vi "Generator.GetEvents.vi"(8 "error in (no error)":errorcluster, 11 "Generator in":refnum<class "Generator.lvclass">) -> (0 "error out":errorcluster, 3 "Generator":cluster{"Public Events":T1, "Public Events":T2})   [LabVIEW 2019, in "Generator.lvclass"]
uses:
  Generator.lvclass
  <vilib>/JKI/JKI SMO/SMO/SMO.lvclass
  Typedefs/PublicEvents--Generator.getGeneratorWaveforms.ctl
  Typedefs/PublicEvents--Cluster.ctl
  <vilib>/JKI/JKI SMO/SMO/Typedefs/Reserve State--Enum.ctl
  <vilib>/JKI/JKI SMO/SMO/Typedefs/SMOState --Enum.ctl
  <vilib>/JKI/JKI SMO/SMO/Typedefs/Public Events.ctl
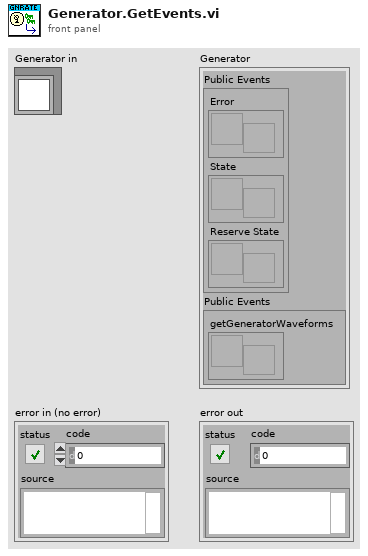
[diagram p1: front panel]
types:
  T1 = typedef "SMO.lvclass/Public Events.ctl" = cluster{"Error":refnum<user-event>, "State":refnum<user-event>, "Reserve State":refnum<user-event>}
  T2 = typedef "Generator.lvclass/PublicEvents--Cluster.ctl" = cluster{"getGeneratorWaveforms":refnum<user-event>}
  T3 = cluster{"Public Events":T1, "Generator.Public Events":T2}
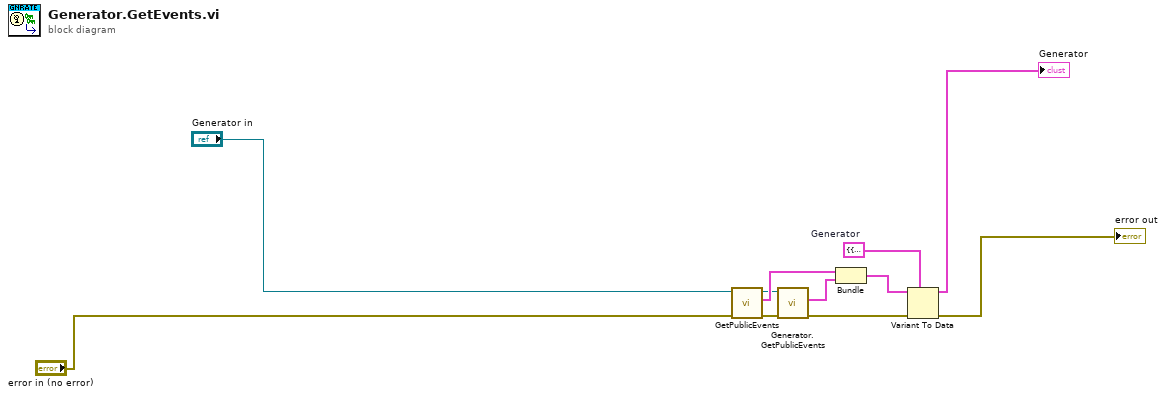
[diagram p0: block diagram]
diagram:
  w8 = cluster{"Public Events":T1, "Public Events":T2} {"Public Events"={"Error"=refnum, "State"=refnum, "Reserve State"=refnum}, "Public Events"={"getGeneratorWaveforms"=refnum}}  # Generator
  n1 = call <vilib>:"GetPublicEvents.vi"("error in (no error)"="error in (no error)", "SMO"="Generator in") -> ("error out"=w4:errorcluster, "Public Events"=w3:T1, "SMO out"=w1:refnum<class "Generator.lvclass">)  [unwired: 7 in]
  n2 = call "Generator.GetPublicEvents.vi"("error in (no error)"=w4, "Generator"=w1) -> ("error out"=w9:errorcluster, "Generator.Public Events"=w5:T2)  [unwired: 7 in, 1 out]
  n3 = Bundle("Public Events"=w3, "Generator.Public Events"=w5) -> (w6:T3)  [unwired: 1 in]
  n4 = Variant To Data(error in=w9, type=w8, Variant=w6) -> (data=→"Generator":cluster{"Public Events":T1, "Public Events":T2}, error out=→"error out":errorcluster)
